vi "NLM.vi"(0 "System no.":i32=1 min=1 max=4 step=1, 2 "Affected axes":string[](array[string]), 3 "Negative soft limit":dbl[](array[numeric]) format="%.6f", 4 "No.of digits":i16=4, 5 "error in":errorcluster) -> (19 "error out":errorcluster)   [LabVIEW 2026]
doc: "Sets negative soft limit for the specified axes. No. of digits is the number of digits after the decimal point in the limit values that will be sent.\n\nE-516, E-517, E-518: The NLM command saves the parameters in RAM only. To save the currently valid parameters to flash ROM, where they become the power-on defaults, you must run WPA.vi. Parameter changes not saved with WPA will be lost when the device is powered off.\n\nE-755: Command not available for E-755.101\n\nE-761: The NLM command saves the parameters in RAM only. To save the currently valid parameters to flash ROM, where they become the power-on defaults, you must run WPA.vi with \"Affected axes\" as an empty array. Parameter changes not saved with WPA will be lost when the E-761 board is powered off or rebooted."
panel:
  # "Sets negative soft limit for the specified axes."
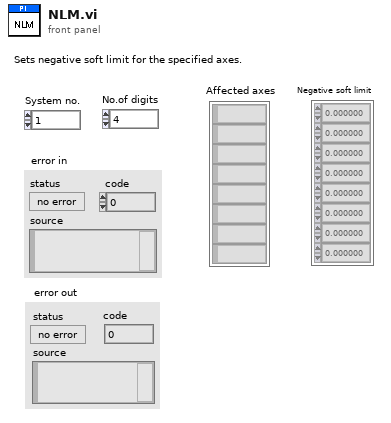
[diagram p1: front panel]
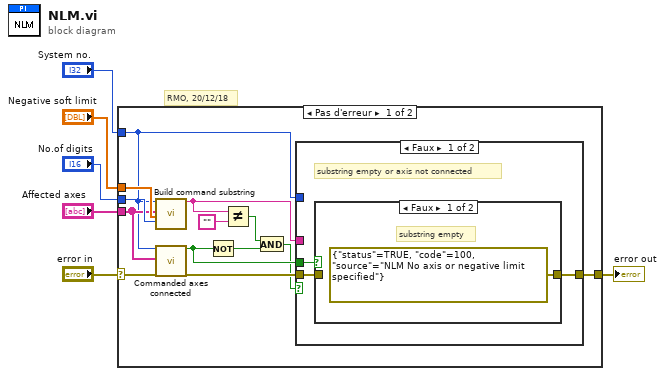
[diagram p0: block diagram]
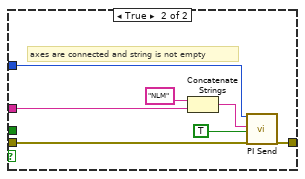
[diagram p3: hidden frame]
diagram:
  # "RMO, 20/12/18"
  n1 = case shown="Pas d'erreur" "error in" {
    selector: "error in" -> [w7 w32]
    tunnel: [w19 w32] -> w6
    tunnel: "Negative soft limit" -> [w16 _]
    tunnel: "No.of digits" -> [w15 _]
    tunnel: "System no." -> [w8 _]
    tunnel: "Affected axes" -> [w13 _]
    frame No Error {
      n2 = call "Build command substring.vi"("System no."=w8, "Affected axes"=w13, "Parameters"=w16, "No. of digits"=w15) -> ("Command substring"=w17:string)  [unwired: 3 in, 12 out]
      n3 = call "Commanded axes connected.vi"("System no."=w8, "Commanded axes"=w13, "error in"=w7) -> ("Controller error"=w11:bool, "error out"=w14:errorcluster)  [unwired: 1 in, 14 out]
      n4 = Not(x=w11) -> (.not. x?=w10:bool)
      n5 = Not Equal?(x=w17, y="") -> (x != y?=w12:bool)
      n6 = And(x=w12, y=w10) -> (x .and. y?=w9:bool)
      n7 = case shown="Faux" w9 {
        tunnel: w17 -> [_ w30]
        tunnel: [w22 w26] -> w19
        tunnel: w14 -> [w20 w27]
        tunnel: w11 -> [w21 _]
        tunnel: w8 -> [_ w25]
        frame False {
          # "substring empty or axis not connected"
          n8 = case shown="Faux" w21 {
            tunnel: [errorcluster {"status"=TRUE, "code"=100, "source"="NLM No axis or negative limit specified"} ("error out") w24] -> w22
            tunnel: w20 -> [_ w24]
            frame False {
              # "substring empty"
            }
            frame True {
              # "commanded axis not connected"
            }
          }
        }
        frame True {
          # "axes are connected and string is not empty"
          n9 = Concatenate Strings("NLM", w30) -> (w28:string)
          n10 = call "PI Send.vi"("System no."=w25, "String to send"=w28, "Attach termination char.?"=TRUE ("Attach Linefeed?"), "error in"=w27) -> ("error out"=w26:errorcluster)  [unwired: 2 in, 13 out]
        }
      }
    }
    frame Error {
    }
  }
  "error out" <- w6
